vi "Validate Configuration Metadata.vi"(8 "error in (no error)":errorcluster) -> (0 "error out":errorcluster, 2 "Invalid Parameters":string, 3 "Is Metadata Valid":bool)   [LabVIEW 2020, in "CancellableMeasurement.lvlib"]
uses:
  CancellableMeasurement.lvlib
  Configuration Metadata.ctl
  TypeDefs/Type Specialization.ctl
  TypeDefs/Key.ctl
  Measurement Configuration.ctl
  b01d6b03-dff1-4d71-9134-3987e39e56b2.vi
  <vilib>/Utility/Data Type/Get Type Definition Path.vi
  <vilib>/Utility/Data Type/NI_Data Type.lvlib
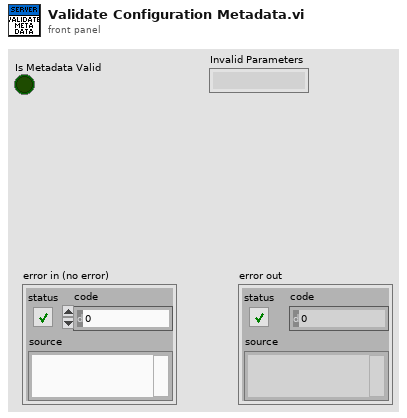
[diagram p1: front panel]
types:
  T1 = typedef "CancellableMeasurement.lvlib/Measurement Configuration.ctl" = cluster{"Array in":dbl[]}
  T2 = typedef "CancellableMeasurement.lvlib/Configuration Metadata.ctl" = cluster{"Parameter Name":string, "Type Specialization":T3, "Annotations":cluster{"Key":T4, "Value":string}[]}[]
  T3 = typedef "CancellableMeasurement.lvlib/Type Specialization.ctl" = enum16{"none", "pin"}
  T4 = typedef "CancellableMeasurement.lvlib/Key.ctl" = enum16{"none", "pin.instrument_type"}
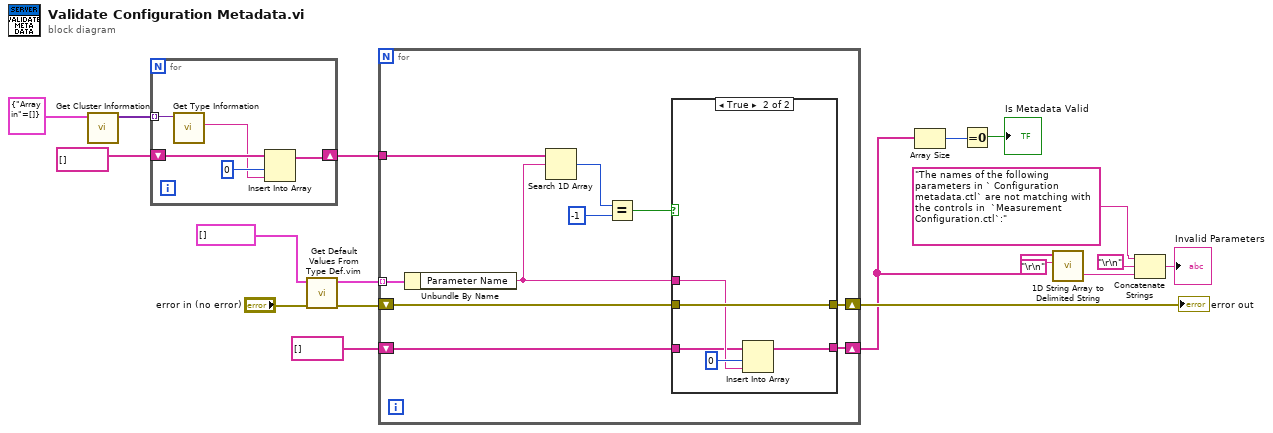
[diagram p0: block diagram]
diagram:
  n1 = call <vilib>:"Get Cluster Information.vi"("variant"=T1 {"Array in"=[]} ("Measurement Configuration")) -> ("cluster elements"=w13:variant[])  [unwired: 9 in, 1 out]
  n2 = for {
    tunnel: w13 -> [w23] mode=indexing
    shift-right: [w19] -> w11
    shift-left: string[] [] -> [w21]
    n3 = call <vilib>:"Get Type Information.vi"("variant"=w23) -> ("name"=w20:string)  [unwired: 6 in, 4 out]
    n4 = Insert Into Array(array=w21, index=0, new element=w20) -> (w19:string[])
  }
  n5 = call "Get Default Values From Type Def.vim"("error in (no error)"="error in (no error)", "Type Def"=T2 [] ("Configuration Metadata")) -> ("error out"=w15:errorcluster, "Default Values"=w16:T2)  [unwired: 8 in]
  n6 = for {
    tunnel: w16 -> [w33] mode=indexing
    shift-right: [w27] -> w9
    shift-left: w15 -> [w28]
    tunnel: w11 -> [w32]
    shift-right: [w24] -> w2
    shift-left: string[] [] -> [w26]
    n7 = Unbundle By Name(w33) -> ("Parameter Name"=w25:string)
    n8 = Search 1D Array(1D array=w32, element=w25) -> (index of element=w31:i32)  [unwired: 1 in]
    n9 = Equal?(x=w31, y=-1) -> (x = y?=w29:bool)
    n10 = case shown="True" w29 {
      tunnel: w28 -> [w35 w40]
      tunnel: [w35 w40] -> w27
      tunnel: w26 -> [w34 w37]
      tunnel: w25 -> [_ w38]
      tunnel: [w34 w36] -> w24
      frame False {
      }
      frame True {
        n11 = Insert Into Array(array=w37, index=0, new element=w38) -> (w36:string[])
      }
    }
  }
  "error out" <- w9
  n12 = Array Size(array=w2) -> (size(s)=w8:i32)
  n13 = Equal To 0?(x=w8) -> (x = 0?=→"Is Metadata Valid":bool)
  n14 = call <vilib>:"1D String Array to Delimited String.vi"("delimiter"="\r\n", "string array"=w2) -> ("delimited string"=w3:string)  [unwired: 9 in]
  n15 = Concatenate Strings("The names of the following parameters in ` Configuration metadata.ctl` are not matching with the controls in  `Measurement Configuration.ctl`:" ("string"), "\r\n", w3) -> (→"Invalid Parameters":string)
